vi "Main.vi"() -> ()   [LabVIEW 2017]
doc: "This template is for the Queued Message Handler design pattern.\n\nThe Event Handling Loop generates messages based on user interface actions.\n\nThe Message Handling Loop processes messages generated by the Event Handling Loop, or by other messages. The messages are string values, so new messages can be added easily to the Message Cases case structure in the Message Handling Loop. Each message cluster can also provide an optional value for Message Data, which is a variant that can be converted to whatever message-specific data is required."
uses:
  controls/UI Data.ctl
  support/Message Queue/Enqueue Message (Single).vi
  <vilib>/Utility/error.llb/Error Cluster From Error Code.vi
  <vilib>/ErrorRing/Error Ring.xnode
  support/Message Queue/Message Queue.lvlib
  support/User Event - Stop/User Event - Stop.lvlib
  logger/logger.lvlib
  server/server.lvlib
  data_processing/data_processing.lvlib
panel:
  out "Status":string
  in  "Exit":bool
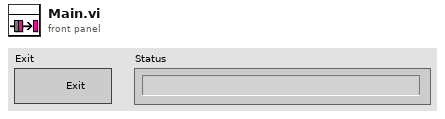
[diagram p1: front panel]
types:
  T1 = typedef "UI Data.ctl" = cluster{"Boolean":bool, "String":string, "Numeric":dbl, "Data Display Ref":refnum<vi>, "Exit Button Ref":refnum<vi>}
  T2 = typedef "Notifiers.ctl" = cluster{"ServerExit":refnum<notifier>, "DataProcessingExit":refnum<notifier>, "WorkerExit":refnum<notifier>}
  T3 = typedef "Message Queue.lvlib/All Message Queues.ctl" = cluster{"MHL":refnum<queue>, "Server":refnum<queue>, "DataProcessing":refnum<queue>, "Worker":refnum<queue>}
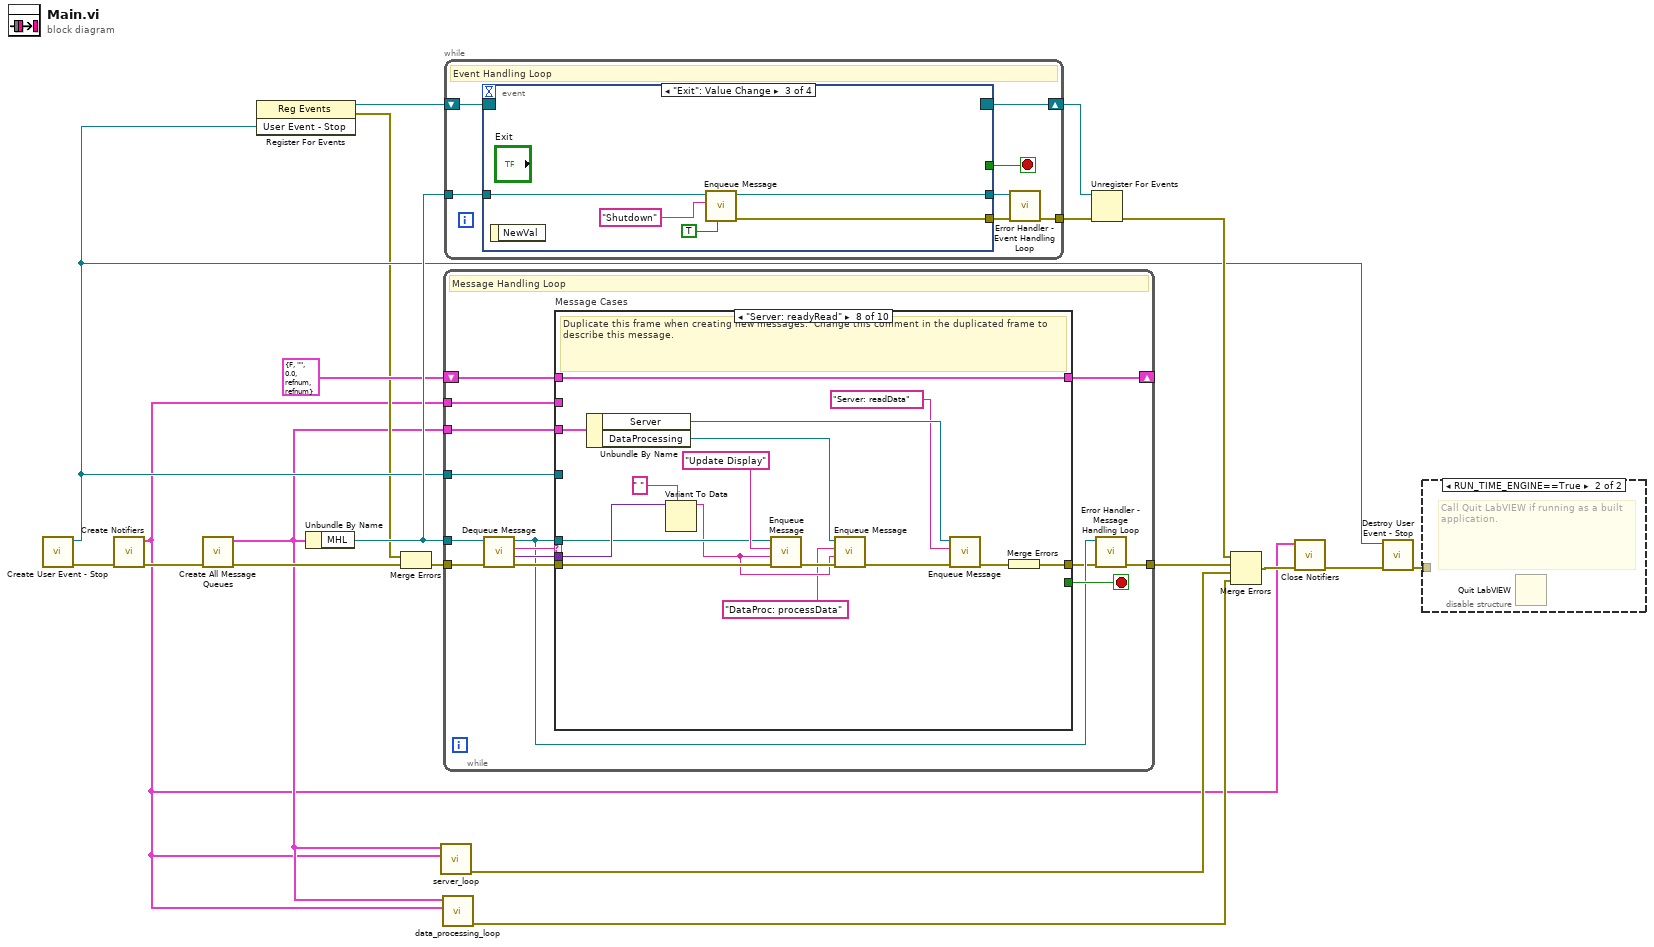
[diagram p0: block diagram]
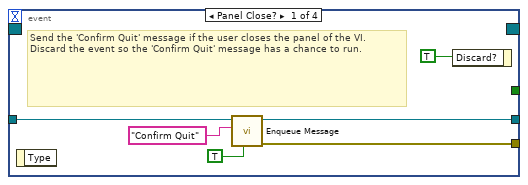
[diagram p3: hidden frame]
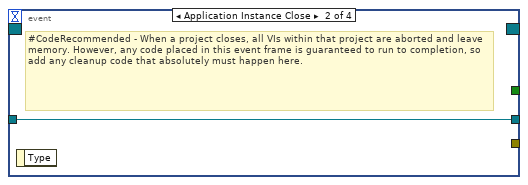
[diagram p4: hidden frame]
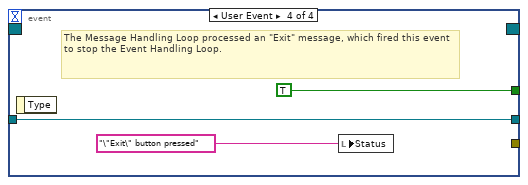
[diagram p5: hidden frame]
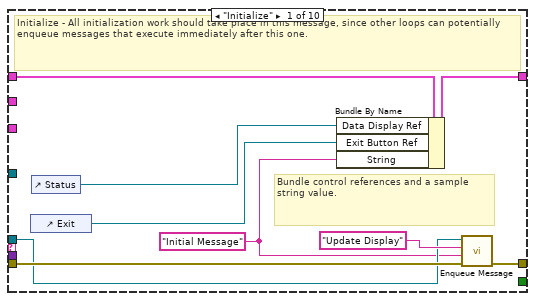
[diagram p6: hidden frame]
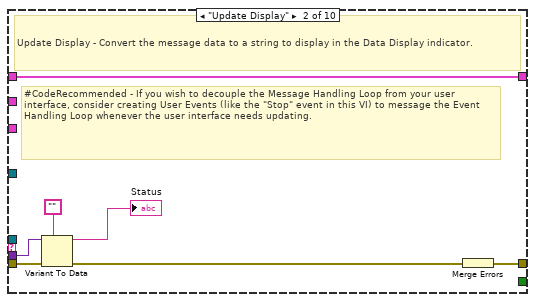
[diagram p7: hidden frame]
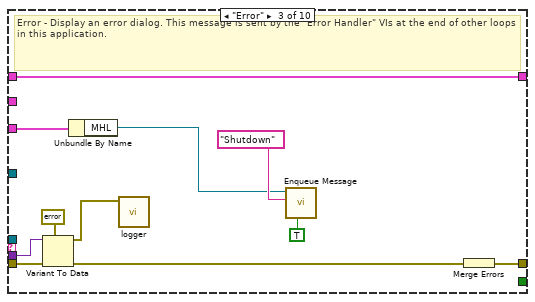
[diagram p8: hidden frame]
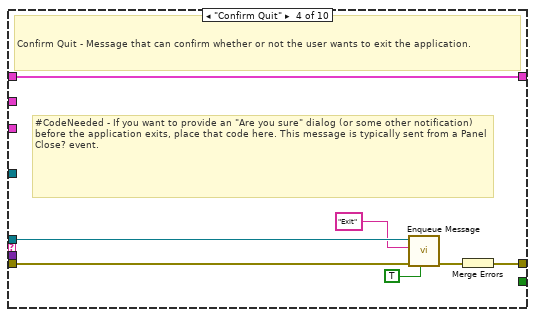
[diagram p9: hidden frame]
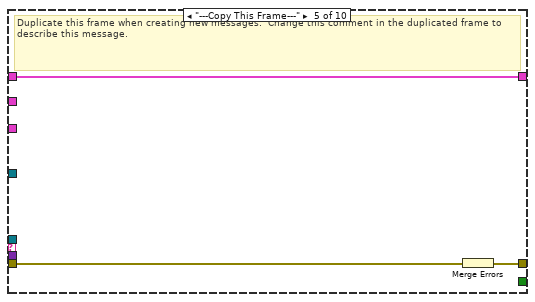
[diagram p10: hidden frame]
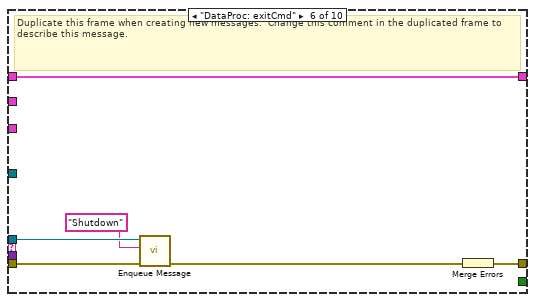
[diagram p11: hidden frame]
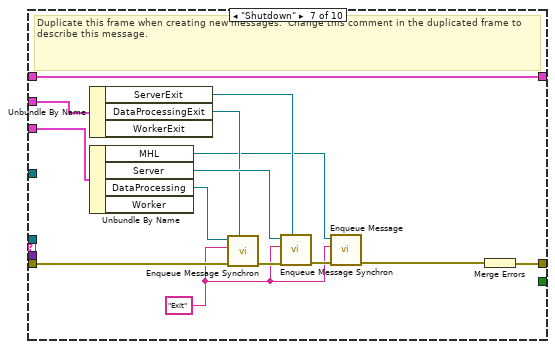
[diagram p12: hidden frame]
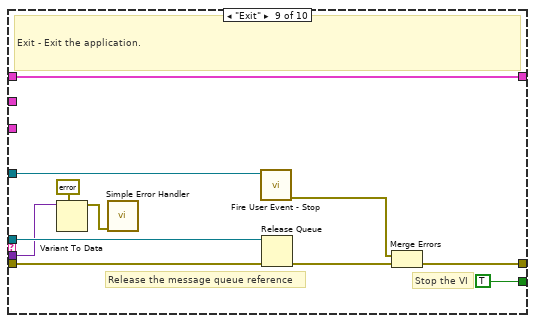
[diagram p13: hidden frame]
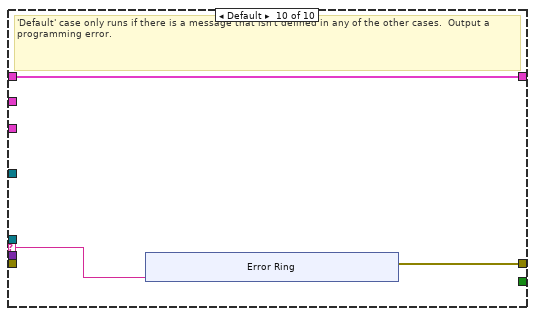
[diagram p14: hidden frame]
diagram:
  n1 = call "Create User Event - Stop.vi"() -> ("error out"=w7:errorcluster, "User Event - Stop"=w11:refnum<user-event>)  [unwired: 10 in]
  n2 = call "Create Notifiers.vi"("error in"=w7) -> ("error out"=w6:errorcluster, "Notifiers"=w1:T2)  [unwired: 9 in]
  n3 = call "Create All Message Queues.vi"("error in (no error)"=w6) -> ("error out"=w20:errorcluster, "Message Queues out"=w5:T3)  [unwired: 9 in]
  n4 = register-events(w11) -> (reference out=w12:refnum<event-registration>, error out=w9:errorcluster)  [unwired: 2 in]
  n5 = Unbundle By Name(w5) -> ("MHL"=w18:refnum<queue>)
  n6 = Merge Errors(w9, w20) -> (w10:errorcluster)
  n7 = call "server_loop.vi"("Notifiers"=w1, "Message Queues"=w5) -> ("error out"=w8:errorcluster)  [unwired: 9 in]
  n8 = call "data_processing_loop.vi"("Notifiers"=w1, "Message Queues"=w5) -> ("error out"=w4:errorcluster)  [unwired: 9 in]
  n9 = while {
    tunnel: w18 -> [w26]
    shift-right: [w33] -> _
    shift-left: T1 {"Boolean"=FALSE, "String"="", "Numeric"=0.0, "Data Display Ref"=refnum, "Exit Button Ref"=refnum} ("Data Cluster") -> [w34]
    tunnel: w11 -> [w31]
    tunnel: w10 -> [w30]
    tunnel: [w24] -> w19
    tunnel: w5 -> [w22]
    tunnel: w1 -> [w21]
    stop <- w32 stop-if-true
    # "Message Handling Loop"
    n10 = call "Dequeue Message.vi"("error in (no error)"=w30, "Message Queue"=w26) -> ("error out"=w29:errorcluster, "Message Data"=w27:variant, "Message"=w28:string, "dup Message Queue"=w25:refnum<queue>)  [unwired: 6 in]
    n11 = case "Message Cases" shown="\"Server: readyRead\"" w28 {
      selector: w28 -> [_ _ _ _ _ _ _ _ _ w119]
      tunnel: w25 -> [w36 _ _ w64 _ w73 _ w101 w118 _]
      tunnel: w29 -> [w42 w48 w61 w68 w71 w75 w87 w103 w111 _]
      tunnel: [w43 w49 w57 w66 w69 w76 w90 w106 w114 w120] -> w23
      tunnel: w34 -> [w41 w50 w60 w67 w70 w77 w91 w107 w117 w121]
      tunnel: [w40 w50 w60 w67 w70 w77 w91 w107 w117 w121] -> w33
      tunnel: [_ _ _ _ _ _ _ _ TRUE _] -> w32
      tunnel: w27 -> [_ w47 w59 _ _ _ _ w105 w108 _]
      tunnel: w31 -> [_ _ _ _ _ _ _ _ w113 _]
      tunnel: w22 -> [_ _ w52 _ _ _ w89 w100 _ _]
      tunnel: w21 -> [_ _ _ _ _ _ w88 _ _ _]
      frame "Initialize" {
        w35 = "Initial Message" ("Initial Message")
        # "Bundle control references and a sample string value."
        # "Initialize - All initialization work should take place in this message, since other loops can potentially enqueue messages that execute immediately after this one."
        n12 = control-ref of="Exit"() -> (w38:refnum<vi>)
        n13 = control-ref of="Status"() -> (w39:refnum<vi>)
        n14 = Bundle By Name(cluster=w41, "Data Display Ref"=w39, "Exit Button Ref"=w38, "String"=w35) -> (w40:T1)
        n15 = call-poly "Enqueue Message.vi"("error in (no error)"=w42, "Message Data"=w35, "Message"="Update Display", "Message Queue"=w36) -> ("error out"=w43:errorcluster)  [unwired: 6 in, 1 out]
      }
      frame "Update Display" {
        # "#CodeRecommended - If you wish to decouple the Message Handling Loop from your user interface, consider creating User Events (like the \"Stop\" event in this VI) to message the Event Handling Loop whenever the user interface needs updating."
        # "Update Display - Convert the message data to a string to display in the Data Display indicator."
        n16 = Variant To Data(error in=w48, type="", Variant=w47) -> (data=→"Status":string, error out=w45:errorcluster)
        n17 = Merge Errors(w45) -> (w49:errorcluster)
      }
      frame "Error" {
        # "Error - Display an error dialog. This message is sent by the \"Error Handler\" VIs at the end of other loops in this application."
        n18 = Variant To Data(error in=w61, type=errorcluster {"status"=FALSE, "code"=0, "source"=""} ("error constant"), Variant=w59) -> (data=w56:errorcluster, error out=w55:errorcluster)
        n19 = Unbundle By Name(w52) -> ("MHL"=w51:refnum<queue>)
        n20 = call "logger.vi"("error in (no error)"=w56) -> ()  [unwired: 11 in]
        n21 = call-poly "Enqueue Message.vi"("Priority Message? (F)"=TRUE, "Message"="Shutdown", "Message Queue"=w51) -> ()  [unwired: 7 in, 2 out]
        n22 = Merge Errors(w55) -> (w57:errorcluster)
      }
      frame "Confirm Quit" {
        # "#CodeNeeded - If you want to provide an \"Are you sure\" dialog (or some other notification) before the application exits, place that code here. This message is typically sent from a Panel Close? event."
        # "Confirm Quit - Message that can confirm whether or not the user wants to exit the application."
        n23 = call-poly "Enqueue Message.vi"("Priority Message? (F)"=TRUE, "error in (no error)"=w68, "Message"="Exit", "Message Queue"=w64) -> ("error out"=w65:errorcluster)  [unwired: 6 in, 1 out]
        n24 = Merge Errors(w65) -> (w66:errorcluster)
      }
      frame "---Copy This Frame---" {
        # "Duplicate this frame when creating new messages.  Change this comment in the duplicated frame to describe this message."
        n25 = Merge Errors(w71) -> (w69:errorcluster)
      }
      frame "DataProc: exitCmd" {
        # "Duplicate this frame when creating new messages.  Change this comment in the duplicated frame to describe this message."
        n26 = call-poly "Enqueue Message.vi"("error in (no error)"=w75, "Message"="Shutdown", "Message Queue"=w73) -> ("error out"=w74:errorcluster)  [unwired: 7 in, 1 out]
        n27 = Merge Errors(w74) -> (w76:errorcluster)
      }
      frame "Shutdown" {
        w78 = "Exit" ("Message")
        # "Duplicate this frame when creating new messages.  Change this comment in the duplicated frame to describe this message."
        n28 = Unbundle By Name(w88) -> ("ServerExit"=w83:refnum<notifier>, "DataProcessingExit"=w84:refnum<notifier>)  [unwired: 1 out]
        n29 = Unbundle By Name(w89) -> ("MHL"=w80:refnum<queue>, "Server"=w85:refnum<queue>, "DataProcessing"=w86:refnum<queue>)  [unwired: 1 out]
        n30 = call "Enqueue Message Synchron.vi"("Notifier"=w84, "error in (no error)"=w87, "Message"=w78, "Message Queue"=w86) -> ("error out"=w82:errorcluster)  [unwired: 6 in, 1 out]
        n31 = call "Enqueue Message Synchron.vi"("Notifier"=w83, "error in (no error)"=w82, "Message"=w78, "Message Queue"=w85) -> ("error out"=w81:errorcluster)  [unwired: 6 in, 1 out]
        n32 = call-poly "Enqueue Message.vi"("error in (no error)"=w81, "Message"=w78, "Message Queue"=w80) -> ("error out"=w79:errorcluster)  [unwired: 7 in, 1 out]
        n33 = Merge Errors(w79) -> (w90:errorcluster)
      }
      frame "Server: readyRead" {
        # "Duplicate this frame when creating new messages.  Change this comment in the duplicated frame to describe this message."
        n34 = Unbundle By Name(w100) -> ("Server"=w99:refnum<queue>, "DataProcessing"=w94:refnum<queue>)
        n35 = Variant To Data(type=" ", Variant=w105) -> (data=w93:string)  [unwired: 1 in, 1 out]
        n36 = call-poly "Enqueue Message.vi"("error in (no error)"=w103, "Message Data"=w93, "Message"="Update Display", "Message Queue"=w101) -> ("error out"=w96:errorcluster)  [unwired: 6 in, 1 out]
        n37 = call-poly "Enqueue Message.vi"("error in (no error)"=w96, "Message Data"=w93, "Message"="DataProc: processData", "Message Queue"=w94) -> ("error out"=w95:errorcluster)  [unwired: 6 in, 1 out]
        n38 = call-poly "Enqueue Message.vi"("error in (no error)"=w95, "Message"="Server: readData", "Message Queue"=w99) -> ("error out"=w97:errorcluster)  [unwired: 7 in, 1 out]
        n39 = Merge Errors(w97) -> (w106:errorcluster)
      }
      frame "Exit" {
        # "Stop the VI"
        # "Release the message queue reference"
        # "Exit - Exit the application."
        n40 = Variant To Data(type=errorcluster {"status"=FALSE, "code"=0, "source"=""} ("error constant"), Variant=w108) -> (data=w109:errorcluster)  [unwired: 1 in, 1 out]
        n41 = call <vilib>:"Simple Error Handler.vi"("error in (no error)"=w109) -> ()  [unwired: 4 in, 5 out]
        n42 = call "Fire User Event - Stop.vi"("User Event - Stop"=w113) -> ("error out"=w112:errorcluster)  [unwired: 10 in]
        n43 = Release Queue(queue=w118, error in (no error)=w111) -> (error out=w115:errorcluster)  [unwired: 1 in, 2 out]
        n44 = Merge Errors(w112, w115) -> (w114:errorcluster)
      }
      frame Default {
        # "'Default' case only runs if there is a message that isn't defined in any of the other cases.  Output a programming error."
        n45 = xnode "Error Ring"("parameter 0"=w119) -> ("error out"=w120:errorcluster)
      }
    }
    n46 = call "Error Handler - Message Handling Loop.vi"("error in (no error)"=w23, "Message Queue"=w25) -> ("dup error in"=w24:errorcluster)  [unwired: 8 in, 1 out]
  }
  n47 = while {
    tunnel: w18 -> [w135]
    shift-right: [w133] -> w16
    shift-left: w12 -> [w134]
    tunnel: [w129] -> w13
    stop <- w131 stop-if-true
    # "Event Handling Loop"
    n48 = event shown="[2] \"Exit\": Value Change" {
      selector: w134 -> [_ _ _ _]
      dyn-events: [_ _ _ _] -> w133
      timeout: _ -> [_ _ _ _]
      tunnel: [_ _ _ TRUE ("Discard?")] -> w131
      tunnel: w135 -> [w140 w142 w147 w150]
      tunnel: [w139 _ w146 _] -> w132
      tunnel: [w138 w142 w145 w150] -> w130
      event Panel Close? {
        # "Send the 'Confirm Quit' message if the user closes the panel of the VI. Discard the event so the 'Confirm Quit' message has a chance to run."
        n49 = event-data() -> ()  [unwired: 1 in, 1 out]
        n50 = call-poly "Enqueue Message.vi"("Priority Message? (F)"=TRUE, "Message"="Confirm Quit", "Message Queue"=w140) -> ("error out"=w139:errorcluster, "dup Message Queue"=w138:refnum<queue>)  [unwired: 7 in]
        n51 = event-data("Discard?"=TRUE) -> ()  [unwired: 1 in, 1 out]
      }
      event Application Instance Close {
        # "#CodeRecommended - When a project closes, all VIs within that project are aborted and leave memory. However, any code placed in this event frame is guaranteed to run to completion, so add any cleanup code that absolutely must happen here."
        n52 = event-data() -> ()  [unwired: 1 in, 1 out]
      }
      event "Exit": Value Change {
        n53 = event-data() -> ()  [unwired: 1 in, 1 out]
        n54 = call-poly "Enqueue Message.vi"("Priority Message? (F)"=TRUE, "Message"="Shutdown", "Message Queue"=w147) -> ("error out"=w146:errorcluster, "dup Message Queue"=w145:refnum<queue>)  [unwired: 7 in]
      }
      event User Event {
        # "The Message Handling Loop processed an \"Exit\" message, which fired this event to stop the Event Handling Loop."
        n55 = event-data() -> ()  [unwired: 1 in, 1 out]
        n56 = local write "Status"("\"Exit\" button pressed" ("VI Stopped")) -> ()
      }
    }
    n57 = call "Error Handler - Event Handling Loop.vi"("error in (no error)"=w132, "Message Queue"=w130) -> ("dup error in"=w129:errorcluster)  [unwired: 8 in, 1 out]
  }
  n58 = Unregister For Events(event registration refnum=w16, error in=w13) -> (error out=w17:errorcluster)
  n59 = Merge Errors(w17, w19, w8, w4) -> (w3:errorcluster)
  n60 = call "Close Notifiers.vi"("error in"=w3, "Notifiers"=w1) -> ("error out"=w2:errorcluster)  [unwired: 9 in]
  n61 = call "Destroy User Event - Stop.vi"("error in (no error)"=w2, "User Event - Stop"=w11) -> ("error out"=w14:errorcluster)  [unwired: 9 in]
  n62 = disable-structure shown="RUN_TIME_ENGINE==True" {
    disable-tunnel: w14 -> [_ _]
    frame condition #0 (active) {
    }
    frame condition #1 {
      # "Call Quit LabVIEW if running as a built application."
      n63 = Quit LabVIEW() -> ()  [unwired: 1 in]
    }
  }
